vi "CheckPosition.vi"(8 "error in":errorcluster, 10 "Car Position":u16(slide) scale=0.0..10.0, 11 "State":string) -> (0 "error out":errorcluster, 3 "Pozycja":bool)   [LabVIEW 2020]
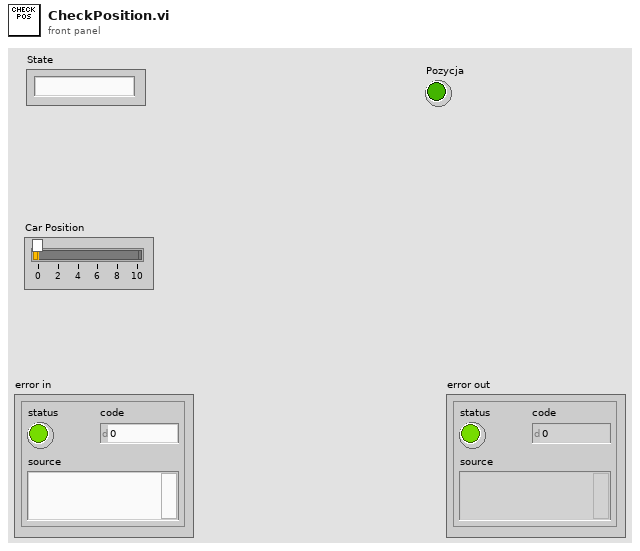
[diagram p1: front panel]
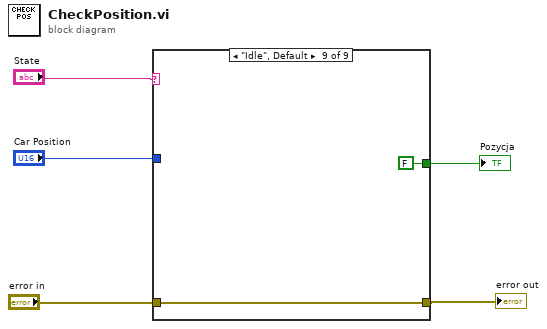
[diagram p0: block diagram]
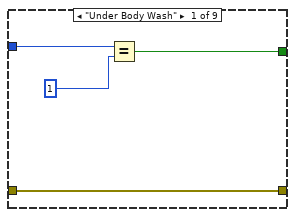
[diagram p2: hidden frame]
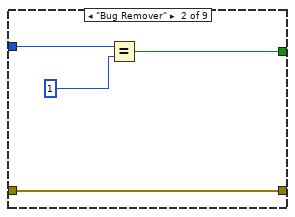
[diagram p3: hidden frame]
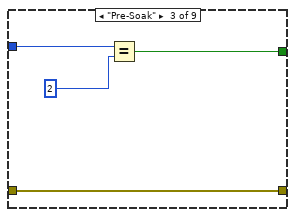
[diagram p4: hidden frame]
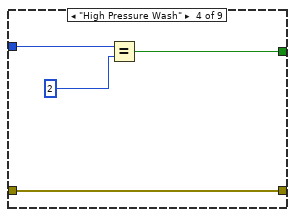
[diagram p5: hidden frame]
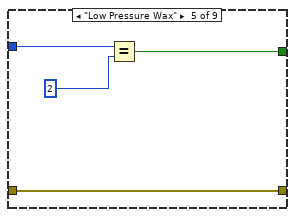
[diagram p6: hidden frame]
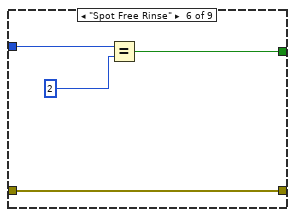
[diagram p7: hidden frame]
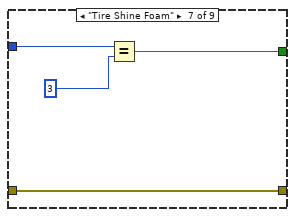
[diagram p8: hidden frame]
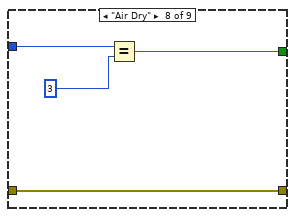
[diagram p9: hidden frame]
diagram:
  n1 = case shown="\"Idle\", Default" "State" {
    tunnel: "Car Position" -> [w8 w12 w16 w20 w24 w28 w32 w36 _]
    tunnel: "error in" -> [w9 w13 w17 w21 w25 w29 w33 w37 w38]
    tunnel: [w9 w13 w17 w21 w25 w29 w33 w37 w38] -> w1
    tunnel: [w6 w10 w14 w18 w22 w26 w30 w34 FALSE] -> w2
    frame "Under Body Wash" {
      n2 = Equal?(x=w8, y=u16 1 ("Car Position")) -> (x = y?=w6:bool)
    }
    frame "Bug Remover" {
      n3 = Equal?(x=w12, y=u16 1 ("Car Position")) -> (x = y?=w10:bool)
    }
    frame "Pre-Soak" {
      n4 = Equal?(x=w16, y=u16 2 ("Car Position")) -> (x = y?=w14:bool)
    }
    frame "High Pressure Wash" {
      n5 = Equal?(x=w20, y=u16 2 ("Car Position")) -> (x = y?=w18:bool)
    }
    frame "Low Pressure Wax" {
      n6 = Equal?(x=w24, y=u16 2 ("Car Position")) -> (x = y?=w22:bool)
    }
    frame "Spot Free Rinse" {
      n7 = Equal?(x=w28, y=u16 2 ("Car Position")) -> (x = y?=w26:bool)
    }
    frame "Tire Shine Foam" {
      n8 = Equal?(x=w32, y=u16 3 ("Car Position")) -> (x = y?=w30:bool)
    }
    frame "Air Dry" {
      n9 = Equal?(x=w36, y=u16 3 ("Car Position")) -> (x = y?=w34:bool)
    }
    frame "Idle", Default {
    }
  }
  "error out" <- w1
  "Pozycja" <- w2
